vi "Get Ethernet Physical Layer Configuration.vi"(8 "error in (no error)":errorcluster, 10 "Configuration (Enable/disable Auto-negotiation of link speed)":i32(ring) items=["Enable/disable Auto-negotiation of link speed", "Set link speed to 10 Base-T or 100 Base T"], 11 "VISA resource name":refnum<visa-resource-name>) -> (0 "error out":errorcluster, 2 "Value":bool, 3 "VISA resource name out":refnum<visa-resource-name>, 4 "Device Errors":cluster{"code":i32, "Text":string}[](array[cluster]))   [LabVIEW 2014, in "Stanford Research DG645 - Driver.lvlib"]
doc: "Interface Command: EPHY? i\nInstrument Error Check\n\nQuery the physical configuration item i. The parameter i may be one of the following:\n\ni Configuration\n0 Auto-negotiation of link speed enabled?\n1 Set link speed to 10 Base-T\n or 100 Base-T\n\nIf auto-negotiation is enabled, the manual link speed selection is ignored. When auto negotiation is disabled, the speed selection manually configured. Due to a bug in the silicon for the microprocessor, the auto-negotiation of link speed can fail. To avoid this bug, the DG645 defaults to manually configured 100 Base-T link speed.\n\nIf Auto-negotiation is disabled, value is false (true otherwise). \n\nIf 10 Base-T is set, value is false (true otherwise)."
uses:
  Stanford Research DG645 - Driver.lvlib
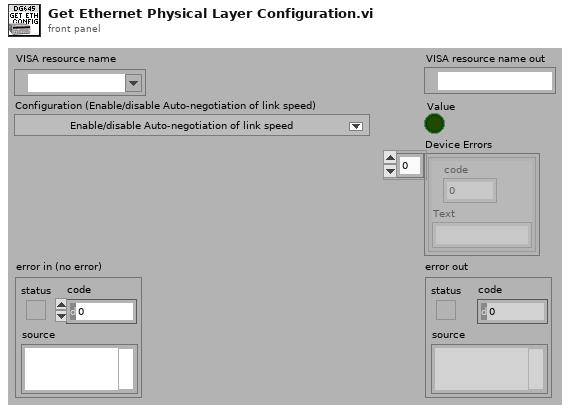
[diagram p1: front panel]
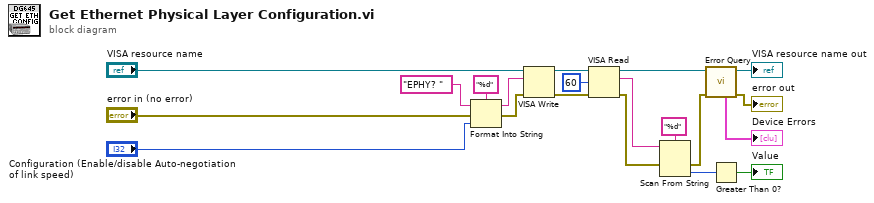
[diagram p0: block diagram]
diagram:
  n1 = Format Into String(format string="%d", initial string="EPHY? " ("command"), error in="error in (no error)", "Configuration (Enable/disable Auto-negotiation of link speed)") -> (resulting string=w4:string, error out=w5:errorcluster)
  n2 = VISA Write(VISA resource name="VISA resource name", write buffer=w4, error in (no error)=w5) -> (VISA resource name out=w12:refnum<visa-resource-name>, error out=w10:errorcluster)  [unwired: 1 out]
  n3 = VISA Read(VISA resource name=w12, byte count=u32 60, error in (no error)=w10) -> (VISA resource name out=w11:refnum<visa-resource-name>, read buffer=w14:string, error out=w13:errorcluster)  [unwired: 1 out]
  n4 = Scan From String(format string="%d", input string=w14, error in=w13) -> (error out=w9:errorcluster, output 1=w2:i32)  [unwired: 2 in, 2 out]
  n5 = call "Error Query.vi"("error in (no error)"=w9, "VISA resource name"=w11) -> ("error out"=→"error out":errorcluster, "VISA resource name out"=→"VISA resource name out":refnum<visa-resource-name>, "Device Errors"=→"Device Errors":cluster{"code":i32, "Text":string}[])  [unwired: 7 in]
  n6 = Greater Than 0?(x=w2) -> (x > 0?=→"Value":bool)
